vi "Default UDP Rigid Joystick.vi"() -> (3 "String":string)   [LabVIEW 2016]
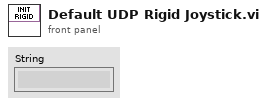
[diagram p1: front panel]
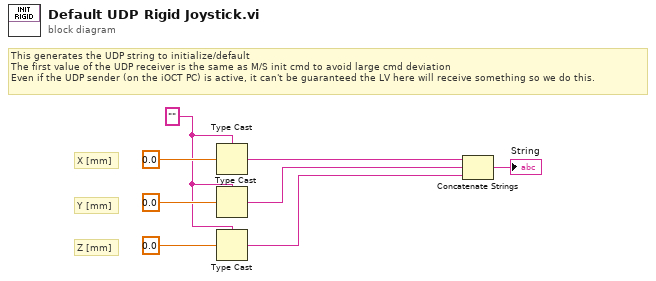
[diagram p0: block diagram]
diagram:
  w4 = "" ("data in")
  # "This generates the UDP string to initialize/default \nThe first value of the UDP receiver is the same as M/S init cmd to avoid large cmd deviation\nEven if the UDP sender (on the iOCT PC) is active, it can't be guaranteed the LV here will receive something so we do this."
  # "Z [mm]"
  # "Y [mm]"
  # "X [mm]"
  n1 = Type Cast(type=w4, x=sgl 0.0 ("number")) -> (*(type *) &x=w1:string)
  n2 = Type Cast(type=w4, x=sgl 0.0 ("number")) -> (*(type *) &x=w3:string)
  n3 = Type Cast(type=w4, x=sgl 0.0 ("number")) -> (*(type *) &x=w2:string)
  n4 = Concatenate Strings(w1, w3, w2) -> (→"String":string)
